vi "Get Chemistries.vi"(0 "reference in":refnum<class "Battery.lvclass">, 5 "Error In":errorcluster) -> (14 "reference out":refnum<class "Battery.lvclass">, 16 "chemistries":string[](array[string]), 19 "Error Out":errorcluster)   [LabVIEW 2023, in "Battery.lvclass"]
uses:
  Battery.lvclass
  Battery.lvclass/Battery.ctl
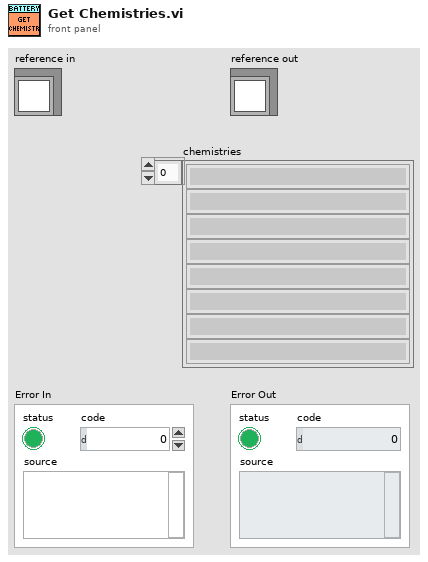
[diagram p1: front panel]
types:
  T1 = typedef "Battery.lvclass/ObjectAttributes.ctl" = cluster{"Python module":path, "Python Session":refnum<k35>, "PybammWrapper":refnum<k38>, "model loaded":bool, "simulation loaded":bool, "simulation enabled":bool, "SOC OCV Curve":dbl[][], "Open Circuit Voltage (V)":dbl, "State of Charge (%)":dbl, "# Cells in Series":u16, "# Cells in Parallel":u16, "Model Parameters":T2, "Simulation Parameters":T3, "Power Module":refnum<class "PowerModuleInterface.lvclass">}
  T2 = typedef "Battery.lvclass/Model Parameters.ctl" = cluster{"chemistry":string, "model_type":string}
  T3 = typedef "Battery.lvclass/Simulation Parameters.ctl" = cluster{"num_rc_pairs":i32, "R0":dbl, "R1":dbl, "C1":dbl, "R2":dbl, "C2":dbl, " nominal_capacity_Ah":dbl, "upper_voltage_cutoff":dbl, "lower_voltage_cutoff":dbl}
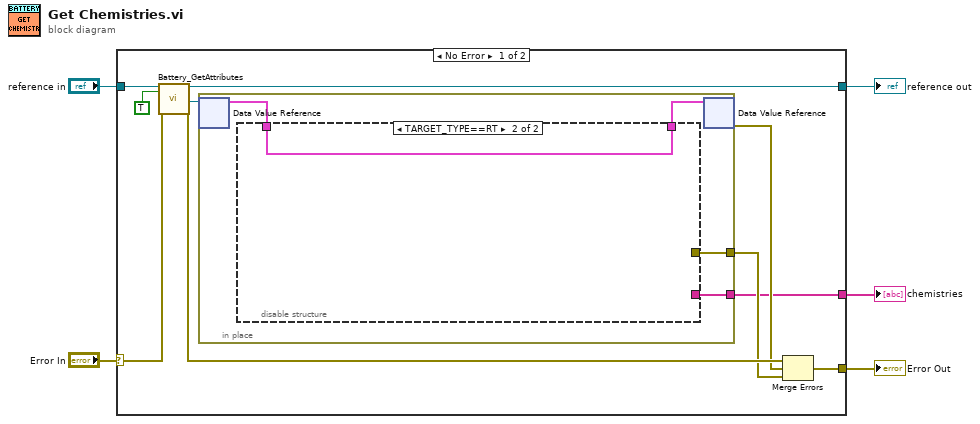
[diagram p0: block diagram]
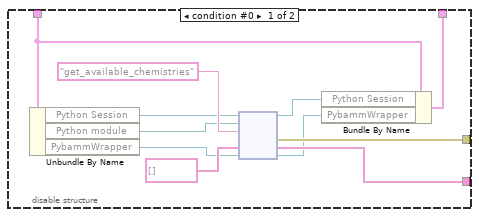
[diagram p2: hidden frame]
diagram:
  n1 = case shown="No Error" "Error In" {
    selector: "Error In" -> [w14 w33]
    tunnel: [w12 w33] -> w4
    tunnel: [w13 w32] -> w2
    tunnel: "reference in" -> [w15 w32]
    tunnel: [w6 _] -> w1
    frame No Error {
      n2 = call "Battery_GetAttributes.vi"("reference in"=w15, "OnlyGetDvrReference(False)"=TRUE, "Error In"=w14) -> ("reference out"=w13:refnum<class "Battery.lvclass">, "DataRef"=w11:refnum<data-value>, "Error Out"=w9:errorcluster)  [unwired: 13 in, 1 out]
      n3 = in-place {
        in-place-border: [w19] -> w7
        in-place-border: [w18] -> w6
        n4 = in-place-dvr #1(w11) -> (w17:T1)  [unwired: 1 out]
        n5 = disable-structure shown="TARGET_TYPE==RT" {
          disable-tunnel: [w25 _] -> w19
          disable-tunnel: [w24 _] -> w18
          disable-tunnel: w17 -> [w23 w31]
          disable-tunnel: [w21 w31] -> w16
          frame condition #0 {
            n6 = Unbundle By Name(w23) -> ("Python Session"=w27:refnum<k35>, "Python module"=w26:path, "PybammWrapper"=w28:refnum<k38>)
            n7 = node(w27, w26, "get_available_chemistries" ("function name"), string[] [], w28) -> (w20:refnum<k35>, w25:errorcluster, w24:string[], w22:refnum<k38>)  [unwired: 1 in, 2 out]
            n8 = Bundle By Name(cluster=w23, "Python Session"=w20, "PybammWrapper"=w22) -> (w21:T1)
          }
          frame condition #1 (active) {
          }
        }
        n9 = in-place-dvr #1(w16) -> (w8:errorcluster)  [unwired: 1 out]
      }
      n10 = Merge Errors(w9, w8, w7) -> (w12:errorcluster)
    }
    frame Error {
    }
  }
  "Error Out" <- w4
  "reference out" <- w2
  "chemistries" <- w1
